vi "5.10 Probabalistic Algorithm 1.vi"(0 "Gains and Parameters":T2={"Control Gain"=0.0, "Line Setpoint in Pixels"=5.0, "Low Pass Gain"=0.0, "Image Low Pass Gain"=0.2, "Line Fullness Setpoint"=0.2, "Line Fullness Std"=0.1, "Max Filter Mod"=-10.0, "Fullness dev"=0.0}, 2 "Buffers Cluster In":T3) -> (3 "Line Def":T5, 4 "Certainty of Line (High is more certain scale is arbitrary)":dbl, 5 "Output Control Signal":dbl, 6 "Buffers Cluster Out":T3)   [LabVIEW 2010]
uses:
  4-High Neurons/4.0-Timing Badass.ctl
  6-OCU Neurons/6.10 Occipital Neurons/6.10.1 LineDef.ctl
  5.10 Buffers Cluster.ctl
  <vilib>/userDefined/High Color/IMAQdx.ctl
  <vilib>/vision/Image Controls.llb/IMAQ Image.ctl
  5.10 Algorithm Parameters and Controls.ctl
panel:
  out "Color Overlay":T1(plugin-control)
  out "Intensity Graph":dbl[][](graph)
  out "B/W Overlay":T1(plugin-control)
  out "Fullness":dbl
  out "Line Aspect Ratio":dbl
  out "Data Sizes":i32[](array[numeric])
  out "Super Heart Beat":T6
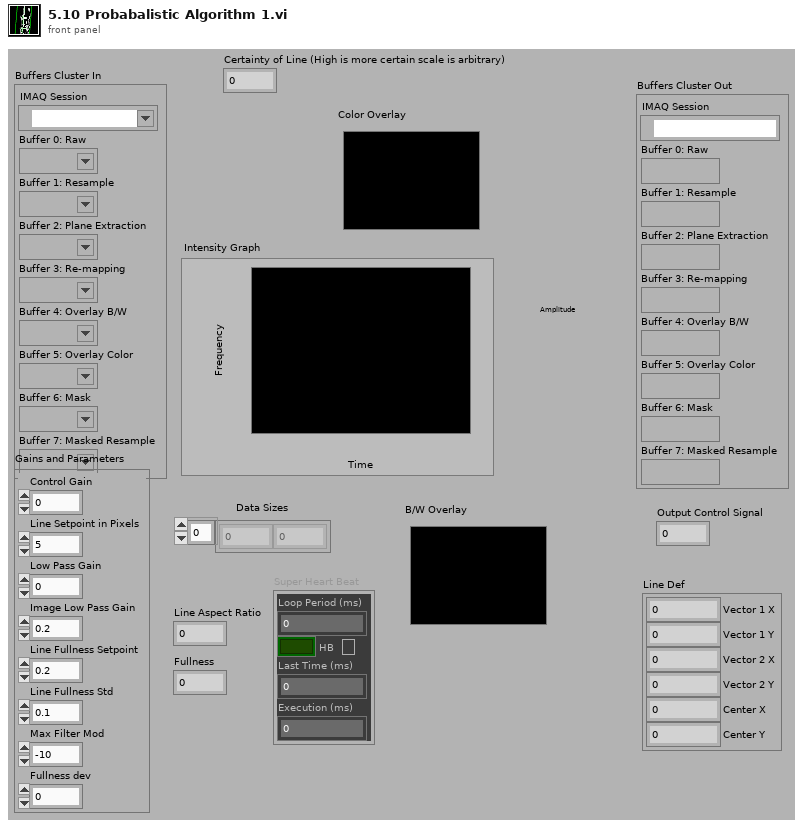
[diagram p1: front panel]
types:
  T1 = typedef "IMAQ Image.ctl" = refnum<image>
  T2 = typedef "5.10 Algorithm Parameters and Controls.ctl" = cluster{"Control Gain":dbl, "Line Setpoint in Pixels":dbl, "Low Pass Gain":dbl, "Image Low Pass Gain":dbl, "Line Fullness Setpoint":dbl, "Line Fullness Std":dbl, "Max Filter Mod":dbl, "Fullness dev":dbl}
  T3 = typedef "5.10 Buffers Cluster.ctl" = cluster{"IMAQ Session":T4, "Buffer 0: Raw":T1, "Buffer 1: Resample":T1, "Buffer 2: Plane Extraction":T1, "Buffer 3: Re-mapping":T1, "Buffer 4: Overlay B/W":T1, "Buffer 5: Overlay Color":T1, "Buffer 6: Mask":T1, "Buffer 7: Masked Resample":T1}
  T4 = typedef "IMAQdx.ctl" = refnum<k21>
  T5 = typedef "6.10.1 LineDef.ctl" = cluster{"Vector 1 X":dbl, "Vector 1 Y":dbl, "Vector 2 X":dbl, "Vector 2 Y":dbl, "Center X":dbl, "Center Y":dbl}
  T6 = typedef "4.0-Timing Badass.ctl" = cluster{"Loop Period (ms)":u32, "HB":bool, "Last Time (ms)":u32, "Execution (ms)":u32}
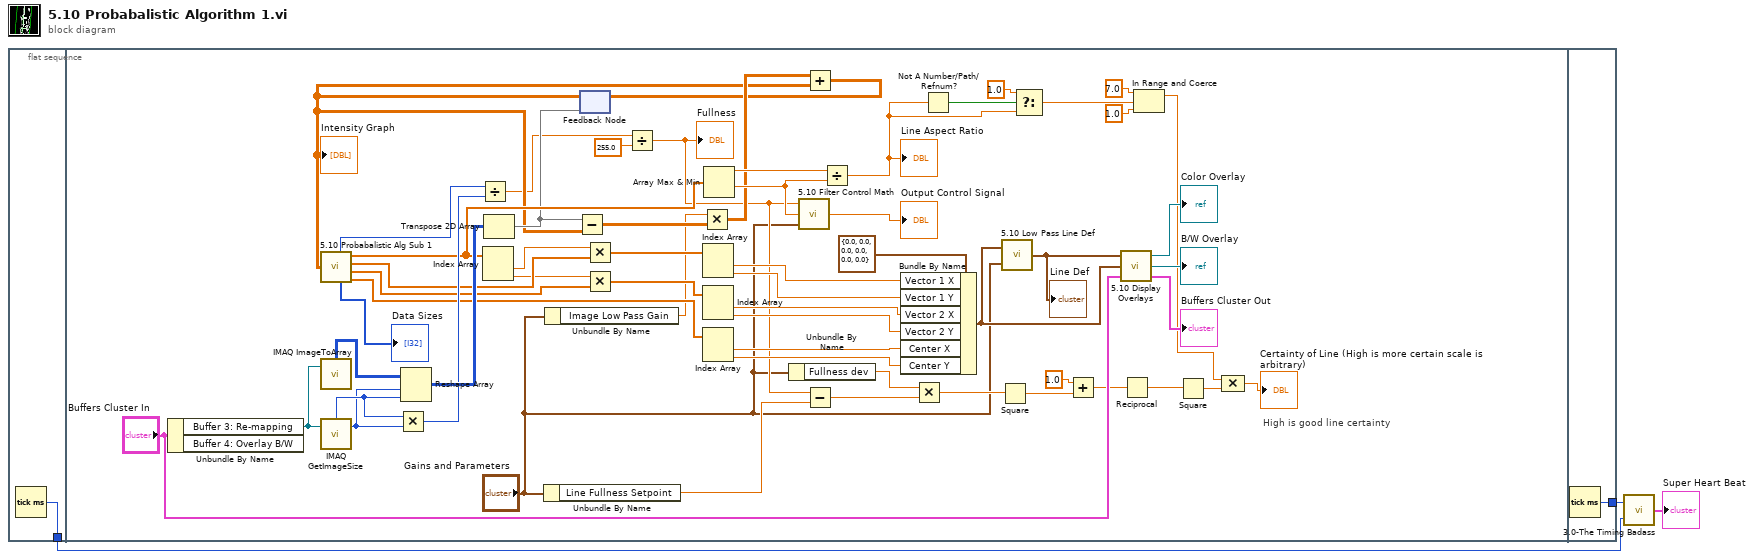
[diagram p0: block diagram]
diagram:
  n1 = flat-sequence {
    tunnel: [w4] -> w2
    tunnel: [w64] -> w3
    frame #0 {
      n2 = Tick Count (ms)() -> (millisecond timer value=w4:u32)
    }
    frame #1 {
      # "High is good line certainty"
      n3 = Unbundle By Name("Buffers Cluster In") -> ("Buffer 3: Re-mapping"=w34:T1)  [unwired: 1 out]
      n4 = call "IMAQ ImageToArray"("Image"=w34) -> ("Image Pixels (U8)"=w53:u8[][])  [unwired: 3 in, 4 out]
      n5 = call "IMAQ GetImageSize"("Image"=w34) -> ("Y Resolution"=w51:i32, "X Resolution"=w52:i32)  [unwired: 3 in, 1 out]
      n6 = Multiply(x=w52, y=w51) -> (x*y=w49:i32)
      n7 = Reshape Array(w53, w51, w52) -> (w62:u8[][])
      n8 = Transpose 2D Array(2D array=w62) -> (transposed array=w36:u8[][])
      n9 = Unbundle By Name("Gains and Parameters") -> ("Line Fullness Setpoint"=w23:dbl)
      n10 = Unbundle By Name("Gains and Parameters") -> ("Image Low Pass Gain"=w24:dbl)
      n11 = feedback #1(w36) -> (w35:dbl[][])
      "Intensity Graph" <- w35
      n12 = call "5.10 Probabalistic Alg Sub 1.vi"("Input Data"=w35) -> ("Pixelsum"=w50:i32, "StdDev"=w42:dbl[], "EigenVector1"=w48:dbl[], "Sizes"=→"Data Sizes":i32[], "EigenVector2"=w47:dbl[], "mean vector"=w44:dbl[])  [unwired: 4 in]
      n13 = Divide(x=w50, y=w49) -> (x/y=w29:dbl)
      n14 = Index Array(array=w42) -> (element #1=w41:dbl, element #2=w40:dbl)  [unwired: 2 in]
      n15 = Subtract(x=w36, y=w35) -> (x-y=w39:dbl[][])
      n16 = Multiply(x=w41, y=w48) -> (x*y=w46:dbl[])
      n17 = Multiply(x=w40, y=w47) -> (x*y=w45:dbl[])
      n18 = Divide(x=w29, y=255.0) -> (x/y=w22:dbl)
      "Fullness" <- w22
      n19 = Multiply(x=w24, y=w39) -> (x*y=w38:dbl[][])
      n20 = Index Array(array=w46) -> (element #1=w59:dbl, element #2=w58:dbl)  [unwired: 2 in]
      n21 = Index Array(array=w45) -> (element #1=w57:dbl, element #2=w56:dbl)  [unwired: 2 in]
      n22 = Index Array(array=w44) -> (element #1=w55:dbl, element #2=w54:dbl)  [unwired: 2 in]
      n23 = Array Max & Min(array=w42) -> (max value=w61:dbl, min value=w43:dbl)  [unwired: 2 out]
      n24 = Unbundle By Name("Gains and Parameters") -> ("Fullness dev"=w5:dbl)
      n25 = call "5.10 Filter Control Math.vi"("Gains and Parameters"="Gains and Parameters", "Lower Std Deviation"=w43, "Fullness"=w22) -> ("Control Output"=→"Output Control Signal":dbl)
      n26 = Add(x=w38, y=w35) -> (x+y=w37:dbl[][])
      n27 = feedback-in #1(w37) -> ()
      n28 = Subtract(x=w22, y=w23) -> (x-y=w21:dbl)
      n29 = Divide(x=w61, y=w43) -> (x/y=w12:dbl)
      "Line Aspect Ratio" <- w12
      n30 = Bundle By Name(cluster=T5 {"Vector 1 X"=0.0, "Vector 1 Y"=0.0, "Vector 2 X"=0.0, "Vector 2 Y"=0.0, "Center X"=0.0, "Center Y"=0.0} ("Line Def"), "Vector 1 X"=w59, "Vector 1 Y"=w58, "Vector 2 X"=w57, "Vector 2 Y"=w56, "Center X"=w55, "Center Y"=w54) -> (w33:T5)
      n31 = Multiply(x=w5, y=w21) -> (x*y=w7:dbl)
      n32 = Not A Number/Path/Refnum?(number/path/refnum=w12) -> (NaN/Path/Refnum?=w10:bool)
      n33 = Square(x=w7) -> (x^2=w20:dbl)
      n34 = call "5.10 Low Pass Line Def.vi"("Gains and Parameters"="Gains and Parameters", "Line Def In"=w33) -> ("Low Pass Line Def Out"=w26:T5)
      "Line Def" <- w26
      n35 = Select(t=1.0, s=w10, f=w12) -> (s? t:f=w11:dbl)
      n36 = Add(x=1.0, y=w20) -> (x+y=w18:dbl)
      n37 = call "5.10 Display Overlays.vi"("Buffers Cluster In"="Buffers Cluster In", "Line Def"=w33, "Low Pass Line Def Out"=w26) -> ("Buffers Cluster In 2"=→"Buffers Cluster Out":T3, "Image Out 2"=→"B/W Overlay":T1, "Image Out"=→"Color Overlay":T1)
      n38 = Reciprocal(x=w18) -> (1/x=w17:dbl)
      n39 = In Range and Coerce(upper limit=7.0, x=w11, lower limit=1.0) -> (coerced(x)=w15:dbl)  [unwired: 1 out]
      n40 = Square(x=w17) -> (x^2=w8:dbl)
      n41 = Compound Arithmetic op=MULTIPLY(w15, w8) -> (→"Certainty of Line (High is more certain scale is arbitrary)":dbl)
    }
    frame #2 {
      n42 = Tick Count (ms)() -> (millisecond timer value=w64:u32)
    }
  }
  n43 = call "3.0-The Timing Badass.vi"("Start"=w2, "End"=w3) -> ("Super Heart Beat"=→"Super Heart Beat":T6)
